vi "HelperRefUID.vi"(0 "Text in":refnum<vi>) -> (1 "UID":i32)   [LabVIEW 2013]
panel:
  out "error out":errorcluster
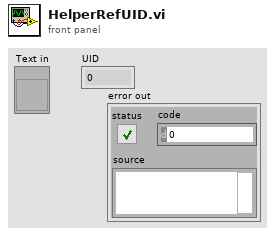
[diagram p1: front panel]
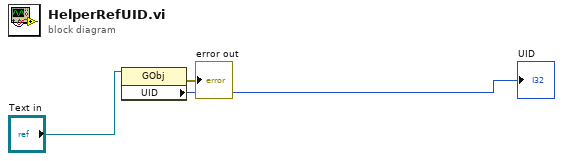
[diagram p0: block diagram]
diagram:
  n1 = property class="GObj"(reference="Text in") -> (error out=→"error out":errorcluster, "UID"=→"UID":i32)  [unwired: 1 in, 1 out]
